vi "Autonomous Independent.vi"() -> ()   [LabVIEW 2019]
doc: "This VI is called when autonomous begins, and will automatically be terminated when autonomous ends. You can carry out timed or sensor driven robot movement independently without needing to return to the caller."
uses:
  <vilib>/Rock Robotics/WPI/Utilities/WPI_GetSetVariantRefNum.vi
  <vilib>/Rock Robotics/Network Tables/NT Read String.vi
  <vilib>/Rock Robotics/Network Tables/NT Write Numeric Array.vi
  <vilib>/Rock Robotics/Network Tables/NT Write Number.vi
  <vilib>/Rock Robotics/Network Tables/NT Write Boolean.vi
  <vilib>/Rock Robotics/WPI/RobotDrive/WPI_RobotDriveArcadeDrive_Standard(NoSaturation).vi
panel:
  out "Current Movement, for debugging":T1 {"Y Joystick Value" scale=1.0..-1.0; "X Joystick Value" scale=-1.0..1.0}
  in  "Array of robot movements":T2(array[cluster])=[{"X Joystick Value"=0.39393939393939403, "Y Joystick Value"=0.0, "Delay (sec)"=1.0, "Movement Name"="turn"}, {"X Joystick Value"=-0.3737373737373737, "Y Joystick Value"=0.0, "Delay (sec)"=1.0, "Movement Name"="turn back"}] {"Y Joystick Value" scale=1.0..-1.0; "X Joystick Value" scale=-1.0..1.0}
  # "Be sure to right-click and choose Data Operations>>Make Current Value default if you want to save the array values with the VI"
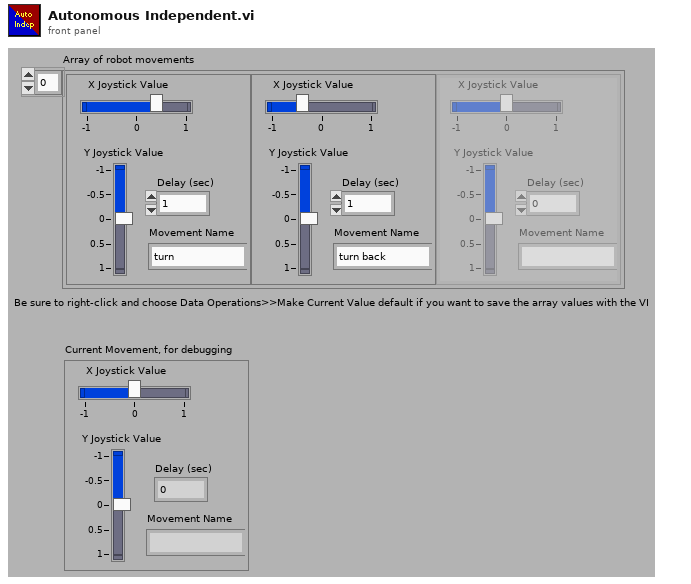
[diagram p1: front panel]
types:
  T1 = cluster{"X Joystick Value":dbl, "Y Joystick Value":dbl, "Delay (sec)":dbl, "Movement Name":string}
  T2 = cluster{"X Joystick Value":dbl, "Y Joystick Value":dbl, "Delay (sec)":dbl, "Movement Name":string}[]
  T3 = typedef "WPI_JoystickDevRef.ctl" = cluster{"Device":T4}
  T4 = typedef "WPI_JoystickDeviceEnum.ctl" = enum16{"USB 0", "USB 1", "USB 2", "USB 3", "USB 4", "USB 5"}
  T5 = typedef "WPI_ServoDeviceRef.ctl" = cluster{"DeviceStatus":errorcluster, "PWM Channel":T6, "DeadBand":T7}
  T6 = typedef "FPGA_DIOPWMChannel.ctl" = enum8{"PWM 0", "PWM 1", "PWM 2", "PWM 3", "PWM 4", "PWM 5", "PWM 6", "PWM 7", "PWM 8", "PWM 9", "PWM MXP 0", "PWM MXP 1", "PWM MXP 2", "PWM MXP 3", "PWM MXP 4", "PWM MXP 5", "PWM MXP 6", "PWM MXP 7", "PWM MXP 8", "PWM MXP 9", "Invalid"}
  T7 = typedef "WPI_PWMDeadband.ctl" = cluster{"Name":string, "maxPositivePwm":i32, "minPositivePwm":i32, "centerPwm":i32, "maxNegativePwm":i32, "minNegativePwm":i32, "angularRange":u16}
  T8 = typedef "WPI_MotorControlDeviceRef.ctl" = cluster{"DeviceStatus":errorcluster, "Type":T9, "PWM":cluster{"PWM Channel":T6, "DeadBand":T7}, "CAN":cluster{"Device Number":u8, "SetOutput VI Ref":variant, "GetOutput VI Ref":variant, "Enable VI Ref":variant, "Disable VI Ref":variant, "Data":variant}, "Invert":bool, "DIO PWM":cluster{"PWM \"Enable\" Channel":T6, "DIOChannel":T10, "PWM Rate":dbl}}
  T9 = typedef "WPI_MotorControlType.ctl" = enum16{"PWM", "CAN", "DIO PWM"}
  T10 = typedef "FPGA_DIOChannel.ctl" = enum8{"DIO 0", "DIO 1", "DIO 2", "DIO 3", "DIO 4", "DIO 5", "DIO 6", "DIO 7", "DIO 8", "DIO 9", "DIO MXP 0", "DIO MXP 1", "DIO MXP 2", "DIO MXP 3", "DIO MXP 4", "DIO MXP 5", "DIO MXP 6", "DIO MXP 7", "DIO MXP 8", "DIO MXP 9", "DIO MXP 10", "DIO MXP 11", "DIO MXP 12", "DIO MXP 13", "DIO MXP 14", "DIO MXP 15", "SPI Port CS1", "SPI Port CS2", "SPI Port CS3", "SPI Port MISO", "SPI Port MOSI", "Invalid"}
  T11 = typedef "WPI_RobotDriveDevRef.ctl" = cluster{"DevStatus":errorcluster, "Motors[]":T8[], "Square Inputs":bool, "Max Output":dbl}
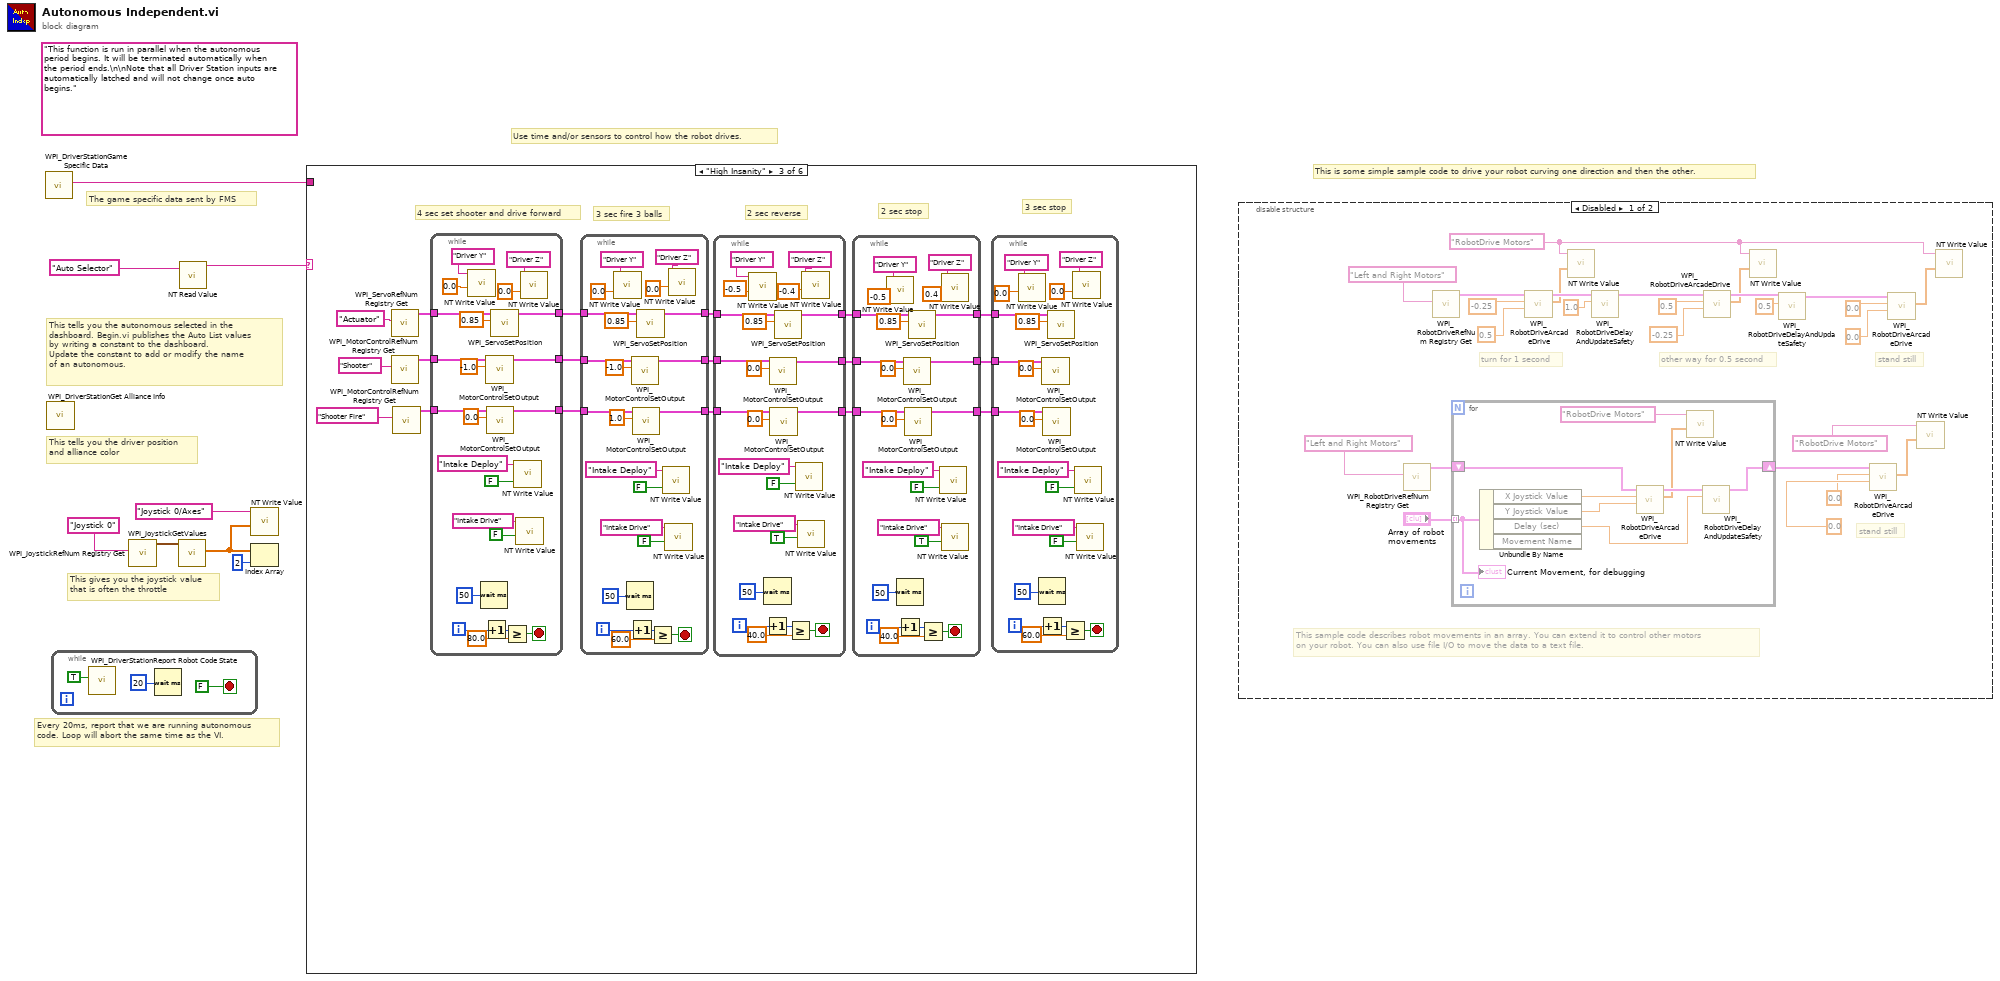
[diagram p0: block diagram]
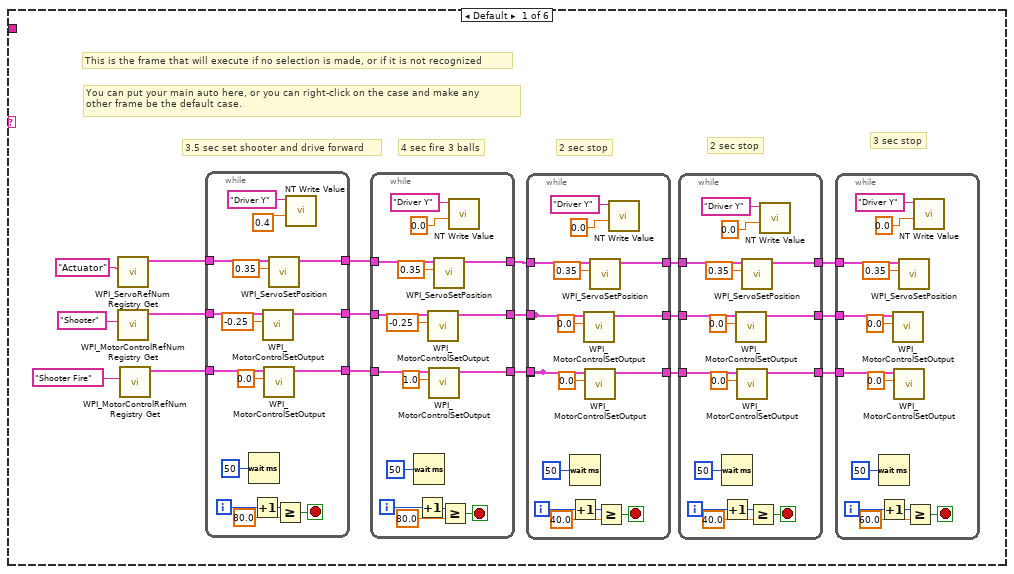
[diagram p3: hidden frame]
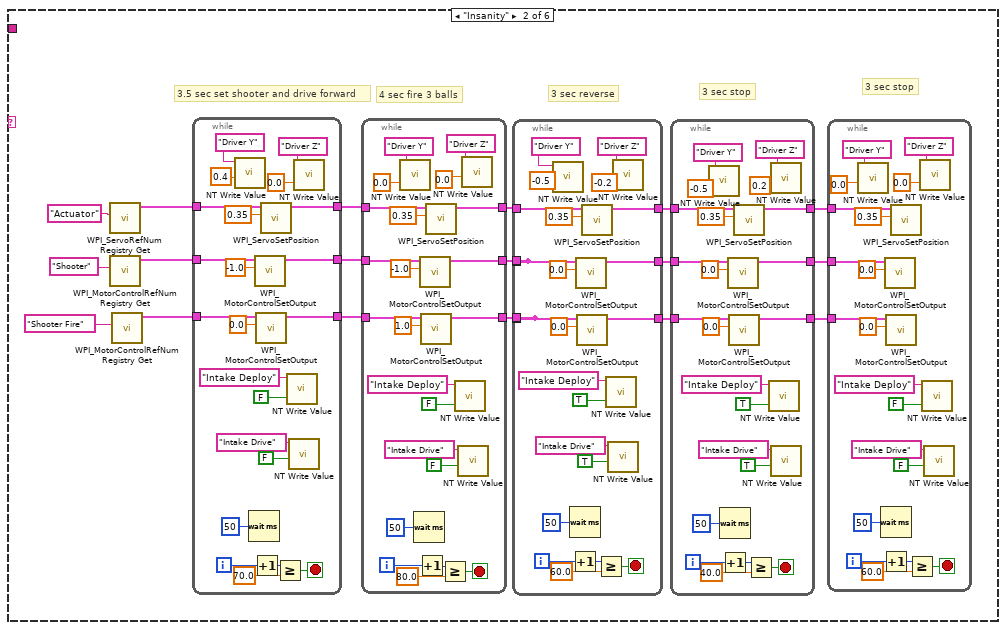
[diagram p4: hidden frame]
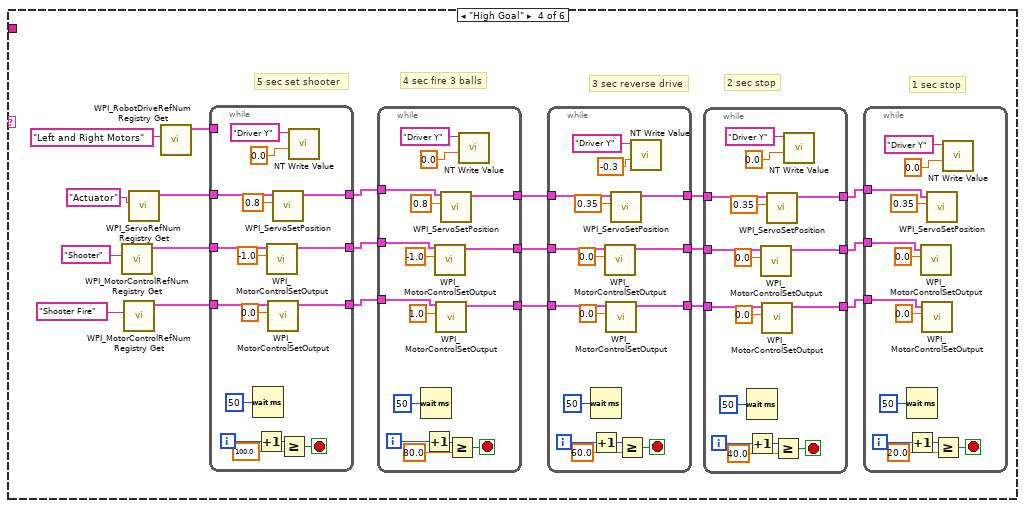
[diagram p5: hidden frame]
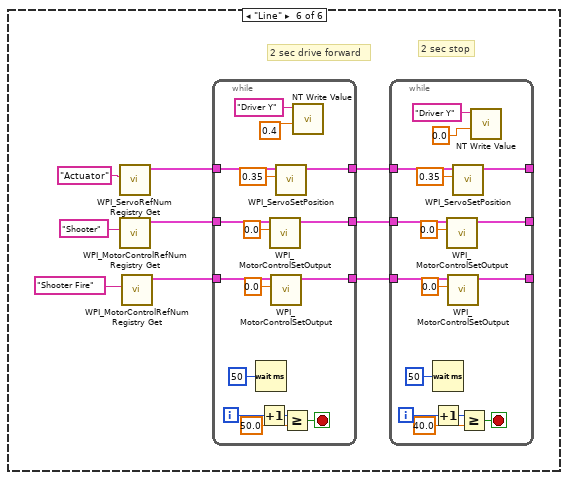
[diagram p7: hidden frame]
diagram:
  (unwired) "This function is run in parallel when the autonomous period begins. It will be terminated automatically when the period ends.\n\nNote that all Driver Station inputs are automatically latched and will not change once auto begins."
  # "This is some simple sample code to drive your robot curving one direction and then the other."
  # "The game specific data sent by FMS"
  # "This tells you the autonomous selected in the \ndashboard. Begin.vi publishes the Auto List values\nby writing a constant to the dashboard.\nUpdate the constant to add or modify the name\nof an autonomous."
  # "Every 20ms, report that we are running autonomous\ncode. Loop will abort the same time as the VI."
  # "This gives you the joystick value\nthat is often the throttle"
  # "Use time and/or sensors to control how the robot drives."
  # "This tells you the driver position\nand alliance color"
  n1 = call <vilib>:"WPI_DriverStationGame Specific Data.vi"() -> ("Game Specific Data"=w1:string)  [unwired: 11 in]
  n2 = call <vilib>:"WPI_DriverStationGet Alliance Info.vi"() -> ()  [unwired: 12 out]
  n3 = while {
    stop <- FALSE stop-if-true
    n4 = call <vilib>:"WPI_DriverStationReport Robot Code State.vi"("Autonomous"=TRUE) -> ()  [unwired: 10 in, 1 out]
    n5 = Wait (ms)(milliseconds to wait=u32 20) -> ()  [unwired: 1 out]
  }
  n6 = call <vilib>:"WPI_JoystickRefNum Registry Get.vi"("refnum name"="Joystick 0") -> ("JoystickDevRef"=w7:T3)  [unwired: 1 in, 9 out]
  n7 = call <vilib>:"WPI_JoystickGetValues.vi"("JoystickDevRef"=w7) -> ("Axes"=w3:dbl[])  [unwired: 6 in, 4 out]
  n8 = call-poly <vilib>:"NT Read Value.vi"("Name"="Auto Selector") -> ("String"=w4:string)  [unwired: 9 in, 1 out]
  n9 = call-poly <vilib>:"NT Write Value.vi"("Numeric Array"=w3, "Name"="Joystick 0/Axes") -> ()  [unwired: 9 in, 1 out]
  n10 = Index Array(array=w3, index=2) -> ()  [unwired: 1 out]
  n11 = case shown="\"High Insanity\"" w4 {
    tunnel: w1 -> [_ _ _ _ _ _]
    frame Default {
      # "2 sec stop"
      # "4 sec fire 3 balls"
      # "3 sec stop"
      # "2 sec stop"
      # "3.5 sec set shooter and drive forward"
      # "You can put your main auto here, or you can right-click on the case and make any\nother frame be the default case."
      # "This is the frame that will execute if no selection is made, or if it is not recognized"
      n12 = call <vilib>:"WPI_ServoRefNum Registry Get.vi"("refnum name"="Actuator") -> ("ServoDeviceRef"=w26:T5)  [unwired: 9 in, 1 out]
      n13 = call <vilib>:"WPI_MotorControlRefNum Registry Get.vi"("refnum name"="Shooter") -> ("MotorControlDevRef"=w25:T8)  [unwired: 9 in, 1 out]
      n14 = call <vilib>:"WPI_MotorControlRefNum Registry Get.vi"("refnum name"="Shooter Fire") -> ("MotorControlDevRef"=w24:T8)  [unwired: 9 in, 1 out]
      n15 = while {
        tunnel: w25 -> [w101]
        tunnel: w24 -> [w100]
        tunnel: w26 -> [w99]
        tunnel: [w95] -> w23
        tunnel: [w94] -> w22
        tunnel: [w93] -> w21
        i -> [w103]
        stop <- w104 stop-if-true
        n16 = Wait (ms)(milliseconds to wait=u32 50) -> ()  [unwired: 1 out]
        n17 = Increment(x=w103) -> (x+1=w102:i32)
        n18 = call <vilib>:"WPI_MotorControlSetOutput.vi"("Output"=-0.25, "MotorControlDevRef"=w101) -> ("MotorControlDevRef"=w94:T8)  [unwired: 7 in, 2 out]
        n19 = call <vilib>:"WPI_MotorControlSetOutput.vi"("Output"=0.0, "MotorControlDevRef"=w100) -> ("MotorControlDevRef"=w93:T8)  [unwired: 7 in, 2 out]
        n20 = call <vilib>:"WPI_ServoSetPosition.vi"("Position"=0.35, "ServoDeviceRef"=w99) -> ("ServoDeviceRef"=w95:T5)  [unwired: 8 in, 1 out]
        n21 = Greater Or Equal?(x=w102, y=80.0) -> (x >= y?=w104:bool)
        n22 = call-poly <vilib>:"NT Write Value.vi"("Numeric"=0.4, "Name"="Driver Y") -> ()  [unwired: 9 in, 1 out]
      }
      n23 = while {
        tunnel: w22 -> [w85]
        tunnel: w21 -> [w84]
        tunnel: w23 -> [w83]
        tunnel: [w79] -> w20
        tunnel: [w78] -> w19
        tunnel: [w77] -> w18
        i -> [w87]
        stop <- w88 stop-if-true
        n24 = Wait (ms)(milliseconds to wait=u32 50) -> ()  [unwired: 1 out]
        n25 = Increment(x=w87) -> (x+1=w86:i32)
        n26 = call <vilib>:"WPI_MotorControlSetOutput.vi"("Output"=-0.25, "MotorControlDevRef"=w85) -> ("MotorControlDevRef"=w78:T8)  [unwired: 7 in, 2 out]
        n27 = call <vilib>:"WPI_MotorControlSetOutput.vi"("Output"=1.0, "MotorControlDevRef"=w84) -> ("MotorControlDevRef"=w77:T8)  [unwired: 7 in, 2 out]
        n28 = call <vilib>:"WPI_ServoSetPosition.vi"("Position"=0.35, "ServoDeviceRef"=w83) -> ("ServoDeviceRef"=w79:T5)  [unwired: 8 in, 1 out]
        n29 = Greater Or Equal?(x=w86, y=80.0) -> (x >= y?=w88:bool)
        n30 = call-poly <vilib>:"NT Write Value.vi"("Numeric"=0.0, "Name"="Driver Y") -> ()  [unwired: 9 in, 1 out]
      }
      n31 = while {
        tunnel: [w60] -> _
        tunnel: [w59] -> _
        tunnel: w20 -> [w69]
        tunnel: [w65] -> w15
        tunnel: [w64] -> w16
        tunnel: [w63] -> w17
        tunnel: w19 -> [w60]
        tunnel: w18 -> [w59]
        i -> [w71]
        stop <- w72 stop-if-true
        n32 = Wait (ms)(milliseconds to wait=u32 50) -> ()  [unwired: 1 out]
        n33 = Increment(x=w71) -> (x+1=w70:i32)
        n34 = call <vilib>:"WPI_MotorControlSetOutput.vi"("Output"=0.0, "MotorControlDevRef"=w60) -> ("MotorControlDevRef"=w64:T8)  [unwired: 7 in, 2 out]
        n35 = call <vilib>:"WPI_MotorControlSetOutput.vi"("Output"=0.0, "MotorControlDevRef"=w59) -> ("MotorControlDevRef"=w63:T8)  [unwired: 7 in, 2 out]
        n36 = call <vilib>:"WPI_ServoSetPosition.vi"("Position"=0.35, "ServoDeviceRef"=w69) -> ("ServoDeviceRef"=w65:T5)  [unwired: 8 in, 1 out]
        n37 = Greater Or Equal?(x=w70, y=40.0) -> (x >= y?=w72:bool)
        n38 = call-poly <vilib>:"NT Write Value.vi"("Numeric"=0.0, "Name"="Driver Y") -> ()  [unwired: 9 in, 1 out]
      }
      n39 = while {
        tunnel: w16 -> [w53]
        tunnel: w17 -> [w52]
        tunnel: w15 -> [w51]
        tunnel: [w47] -> w14
        tunnel: [w46] -> w13
        tunnel: [w45] -> w12
        i -> [w55]
        stop <- w56 stop-if-true
        n40 = Wait (ms)(milliseconds to wait=u32 50) -> ()  [unwired: 1 out]
        n41 = Increment(x=w55) -> (x+1=w54:i32)
        n42 = call <vilib>:"WPI_MotorControlSetOutput.vi"("Output"=0.0, "MotorControlDevRef"=w53) -> ("MotorControlDevRef"=w46:T8)  [unwired: 7 in, 2 out]
        n43 = call <vilib>:"WPI_MotorControlSetOutput.vi"("Output"=0.0, "MotorControlDevRef"=w52) -> ("MotorControlDevRef"=w45:T8)  [unwired: 7 in, 2 out]
        n44 = call <vilib>:"WPI_ServoSetPosition.vi"("Position"=0.35, "ServoDeviceRef"=w51) -> ("ServoDeviceRef"=w47:T5)  [unwired: 8 in, 1 out]
        n45 = Greater Or Equal?(x=w54, y=40.0) -> (x >= y?=w56:bool)
        n46 = call-poly <vilib>:"NT Write Value.vi"("Numeric"=0.0, "Name"="Driver Y") -> ()  [unwired: 9 in, 1 out]
      }
      n47 = while {
        tunnel: w13 -> [w37]
        tunnel: w12 -> [w36]
        tunnel: w14 -> [w35]
        i -> [w39]
        stop <- w40 stop-if-true
        n48 = Wait (ms)(milliseconds to wait=u32 50) -> ()  [unwired: 1 out]
        n49 = Increment(x=w39) -> (x+1=w38:i32)
        n50 = call <vilib>:"WPI_MotorControlSetOutput.vi"("Output"=0.0, "MotorControlDevRef"=w37) -> ()  [unwired: 7 in, 3 out]
        n51 = call <vilib>:"WPI_MotorControlSetOutput.vi"("Output"=0.0, "MotorControlDevRef"=w36) -> ()  [unwired: 7 in, 3 out]
        n52 = call <vilib>:"WPI_ServoSetPosition.vi"("Position"=0.35, "ServoDeviceRef"=w35) -> ()  [unwired: 8 in, 2 out]
        n53 = Greater Or Equal?(x=w38, y=60.0) -> (x >= y?=w40:bool)
        n54 = call-poly <vilib>:"NT Write Value.vi"("Numeric"=0.0, "Name"="Driver Y") -> ()  [unwired: 9 in, 1 out]
      }
    }
    frame "Insanity" {
      # "3 sec reverse"
      # "4 sec fire 3 balls"
      # "3 sec stop"
      # "3 sec stop"
      # "3.5 sec set shooter and drive forward"
      n55 = call <vilib>:"WPI_ServoRefNum Registry Get.vi"("refnum name"="Actuator") -> ("ServoDeviceRef"=w121:T5)  [unwired: 9 in, 1 out]
      n56 = call <vilib>:"WPI_MotorControlRefNum Registry Get.vi"("refnum name"="Shooter") -> ("MotorControlDevRef"=w120:T8)  [unwired: 9 in, 1 out]
      n57 = call <vilib>:"WPI_MotorControlRefNum Registry Get.vi"("refnum name"="Shooter Fire") -> ("MotorControlDevRef"=w119:T8)  [unwired: 9 in, 1 out]
      n58 = while {
        tunnel: w120 -> [w226]
        tunnel: w119 -> [w225]
        tunnel: w121 -> [w224]
        tunnel: [w220] -> w118
        tunnel: [w219] -> w117
        tunnel: [w218] -> w116
        i -> [w228]
        stop <- w229 stop-if-true
        n59 = call-poly <vilib>:"NT Write Value.vi"("Numeric"=0.4, "Name"="Driver Y") -> ()  [unwired: 9 in, 1 out]
        n60 = Wait (ms)(milliseconds to wait=u32 50) -> ()  [unwired: 1 out]
        n61 = Increment(x=w228) -> (x+1=w227:i32)
        n62 = call <vilib>:"WPI_MotorControlSetOutput.vi"("Output"=-1.0, "MotorControlDevRef"=w226) -> ("MotorControlDevRef"=w219:T8)  [unwired: 7 in, 2 out]
        n63 = call <vilib>:"WPI_MotorControlSetOutput.vi"("Output"=0.0, "MotorControlDevRef"=w225) -> ("MotorControlDevRef"=w218:T8)  [unwired: 7 in, 2 out]
        n64 = call <vilib>:"WPI_ServoSetPosition.vi"("Position"=0.35, "ServoDeviceRef"=w224) -> ("ServoDeviceRef"=w220:T5)  [unwired: 8 in, 1 out]
        n65 = Greater Or Equal?(x=w227, y=70.0) -> (x >= y?=w229:bool)
        n66 = call-poly <vilib>:"NT Write Value.vi"("Boolean"=FALSE, "Name"="Intake Deploy") -> ()  [unwired: 9 in, 1 out]
        n67 = call-poly <vilib>:"NT Write Value.vi"("Boolean"=FALSE, "Name"="Intake Drive") -> ()  [unwired: 9 in, 1 out]
        n68 = call-poly <vilib>:"NT Write Value.vi"("Numeric"=0.0, "Name"="Driver Z") -> ()  [unwired: 9 in, 1 out]
      }
      n69 = while {
        tunnel: w117 -> [w204]
        tunnel: w116 -> [w203]
        tunnel: w118 -> [w202]
        tunnel: [w198] -> w115
        tunnel: [w197] -> w114
        tunnel: [w196] -> w113
        i -> [w206]
        stop <- w207 stop-if-true
        n70 = call-poly <vilib>:"NT Write Value.vi"("Numeric"=0.0, "Name"="Driver Y") -> ()  [unwired: 9 in, 1 out]
        n71 = Wait (ms)(milliseconds to wait=u32 50) -> ()  [unwired: 1 out]
        n72 = Increment(x=w206) -> (x+1=w205:i32)
        n73 = call <vilib>:"WPI_MotorControlSetOutput.vi"("Output"=-1.0, "MotorControlDevRef"=w204) -> ("MotorControlDevRef"=w197:T8)  [unwired: 7 in, 2 out]
        n74 = call <vilib>:"WPI_MotorControlSetOutput.vi"("Output"=1.0, "MotorControlDevRef"=w203) -> ("MotorControlDevRef"=w196:T8)  [unwired: 7 in, 2 out]
        n75 = call <vilib>:"WPI_ServoSetPosition.vi"("Position"=0.35, "ServoDeviceRef"=w202) -> ("ServoDeviceRef"=w198:T5)  [unwired: 8 in, 1 out]
        n76 = Greater Or Equal?(x=w205, y=80.0) -> (x >= y?=w207:bool)
        n77 = call-poly <vilib>:"NT Write Value.vi"("Boolean"=FALSE, "Name"="Intake Deploy") -> ()  [unwired: 9 in, 1 out]
        n78 = call-poly <vilib>:"NT Write Value.vi"("Boolean"=FALSE, "Name"="Intake Drive") -> ()  [unwired: 9 in, 1 out]
        n79 = call-poly <vilib>:"NT Write Value.vi"("Numeric"=0.0, "Name"="Driver Z") -> ()  [unwired: 9 in, 1 out]
      }
      n80 = while {
        tunnel: [w173] -> _
        tunnel: [w172] -> _
        tunnel: w115 -> [w182]
        tunnel: [w178] -> w110
        tunnel: [w177] -> w111
        tunnel: [w176] -> w112
        tunnel: w114 -> [w173]
        tunnel: w113 -> [w172]
        i -> [w184]
        stop <- w185 stop-if-true
        n81 = call-poly <vilib>:"NT Write Value.vi"("Numeric"=-0.5, "Name"="Driver Y") -> ()  [unwired: 9 in, 1 out]
        n82 = Wait (ms)(milliseconds to wait=u32 50) -> ()  [unwired: 1 out]
        n83 = Increment(x=w184) -> (x+1=w183:i32)
        n84 = call <vilib>:"WPI_MotorControlSetOutput.vi"("Output"=0.0, "MotorControlDevRef"=w173) -> ("MotorControlDevRef"=w177:T8)  [unwired: 7 in, 2 out]
        n85 = call <vilib>:"WPI_MotorControlSetOutput.vi"("Output"=0.0, "MotorControlDevRef"=w172) -> ("MotorControlDevRef"=w176:T8)  [unwired: 7 in, 2 out]
        n86 = call <vilib>:"WPI_ServoSetPosition.vi"("Position"=0.35, "ServoDeviceRef"=w182) -> ("ServoDeviceRef"=w178:T5)  [unwired: 8 in, 1 out]
        n87 = Greater Or Equal?(x=w183, y=60.0) -> (x >= y?=w185:bool)
        n88 = call-poly <vilib>:"NT Write Value.vi"("Boolean"=TRUE, "Name"="Intake Deploy") -> ()  [unwired: 9 in, 1 out]
        n89 = call-poly <vilib>:"NT Write Value.vi"("Boolean"=TRUE, "Name"="Intake Drive") -> ()  [unwired: 9 in, 1 out]
        n90 = call-poly <vilib>:"NT Write Value.vi"("Numeric"=-0.2, "Name"="Driver Z") -> ()  [unwired: 9 in, 1 out]
      }
      n91 = while {
        tunnel: w111 -> [w160]
        tunnel: w112 -> [w159]
        tunnel: w110 -> [w158]
        tunnel: [w154] -> w109
        tunnel: [w153] -> w108
        tunnel: [w152] -> w107
        i -> [w162]
        stop <- w163 stop-if-true
        n92 = call-poly <vilib>:"NT Write Value.vi"("Numeric"=-0.5, "Name"="Driver Y") -> ()  [unwired: 9 in, 1 out]
        n93 = Wait (ms)(milliseconds to wait=u32 50) -> ()  [unwired: 1 out]
        n94 = Increment(x=w162) -> (x+1=w161:i32)
        n95 = call <vilib>:"WPI_MotorControlSetOutput.vi"("Output"=0.0, "MotorControlDevRef"=w160) -> ("MotorControlDevRef"=w153:T8)  [unwired: 7 in, 2 out]
        n96 = call <vilib>:"WPI_MotorControlSetOutput.vi"("Output"=0.0, "MotorControlDevRef"=w159) -> ("MotorControlDevRef"=w152:T8)  [unwired: 7 in, 2 out]
        n97 = call <vilib>:"WPI_ServoSetPosition.vi"("Position"=0.35, "ServoDeviceRef"=w158) -> ("ServoDeviceRef"=w154:T5)  [unwired: 8 in, 1 out]
        n98 = Greater Or Equal?(x=w161, y=40.0) -> (x >= y?=w163:bool)
        n99 = call-poly <vilib>:"NT Write Value.vi"("Boolean"=TRUE, "Name"="Intake Deploy") -> ()  [unwired: 9 in, 1 out]
        n100 = call-poly <vilib>:"NT Write Value.vi"("Numeric"=0.2, "Name"="Driver Z") -> ()  [unwired: 9 in, 1 out]
        n101 = call-poly <vilib>:"NT Write Value.vi"("Boolean"=TRUE, "Name"="Intake Drive") -> ()  [unwired: 9 in, 1 out]
      }
      n102 = while {
        tunnel: w108 -> [w138]
        tunnel: w107 -> [w137]
        tunnel: w109 -> [w136]
        i -> [w140]
        stop <- w141 stop-if-true
        n103 = call-poly <vilib>:"NT Write Value.vi"("Numeric"=0.0, "Name"="Driver Y") -> ()  [unwired: 9 in, 1 out]
        n104 = Wait (ms)(milliseconds to wait=u32 50) -> ()  [unwired: 1 out]
        n105 = Increment(x=w140) -> (x+1=w139:i32)
        n106 = call <vilib>:"WPI_MotorControlSetOutput.vi"("Output"=0.0, "MotorControlDevRef"=w138) -> ()  [unwired: 7 in, 3 out]
        n107 = call <vilib>:"WPI_MotorControlSetOutput.vi"("Output"=0.0, "MotorControlDevRef"=w137) -> ()  [unwired: 7 in, 3 out]
        n108 = call <vilib>:"WPI_ServoSetPosition.vi"("Position"=0.35, "ServoDeviceRef"=w136) -> ()  [unwired: 8 in, 2 out]
        n109 = Greater Or Equal?(x=w139, y=60.0) -> (x >= y?=w141:bool)
        n110 = call-poly <vilib>:"NT Write Value.vi"("Numeric"=0.0, "Name"="Driver Z") -> ()  [unwired: 9 in, 1 out]
        n111 = call-poly <vilib>:"NT Write Value.vi"("Boolean"=FALSE, "Name"="Intake Deploy") -> ()  [unwired: 9 in, 1 out]
        n112 = call-poly <vilib>:"NT Write Value.vi"("Boolean"=FALSE, "Name"="Intake Drive") -> ()  [unwired: 9 in, 1 out]
      }
    }
    frame "High Insanity" {
      # "2 sec reverse"
      # "3 sec fire 3 balls"
      # "3 sec stop"
      # "2 sec stop"
      # "4 sec set shooter and drive forward"
      n113 = call <vilib>:"WPI_ServoRefNum Registry Get.vi"("refnum name"="Actuator") -> ("ServoDeviceRef"=w246:T5)  [unwired: 9 in, 1 out]
      n114 = call <vilib>:"WPI_MotorControlRefNum Registry Get.vi"("refnum name"="Shooter") -> ("MotorControlDevRef"=w245:T8)  [unwired: 9 in, 1 out]
      n115 = call <vilib>:"WPI_MotorControlRefNum Registry Get.vi"("refnum name"="Shooter Fire") -> ("MotorControlDevRef"=w244:T8)  [unwired: 9 in, 1 out]
      n116 = while {
        tunnel: w245 -> [w351]
        tunnel: w244 -> [w350]
        tunnel: w246 -> [w349]
        tunnel: [w345] -> w243
        tunnel: [w344] -> w242
        tunnel: [w343] -> w241
        i -> [w353]
        stop <- w354 stop-if-true
        n117 = call-poly <vilib>:"NT Write Value.vi"("Numeric"=0.0, "Name"="Driver Y") -> ()  [unwired: 9 in, 1 out]
        n118 = Wait (ms)(milliseconds to wait=u32 50) -> ()  [unwired: 1 out]
        n119 = Increment(x=w353) -> (x+1=w352:i32)
        n120 = call <vilib>:"WPI_MotorControlSetOutput.vi"("Output"=-1.0, "MotorControlDevRef"=w351) -> ("MotorControlDevRef"=w344:T8)  [unwired: 7 in, 2 out]
        n121 = call <vilib>:"WPI_MotorControlSetOutput.vi"("Output"=0.0, "MotorControlDevRef"=w350) -> ("MotorControlDevRef"=w343:T8)  [unwired: 7 in, 2 out]
        n122 = call <vilib>:"WPI_ServoSetPosition.vi"("Position"=0.85, "ServoDeviceRef"=w349) -> ("ServoDeviceRef"=w345:T5)  [unwired: 8 in, 1 out]
        n123 = Greater Or Equal?(x=w352, y=80.0) -> (x >= y?=w354:bool)
        n124 = call-poly <vilib>:"NT Write Value.vi"("Boolean"=FALSE, "Name"="Intake Deploy") -> ()  [unwired: 9 in, 1 out]
        n125 = call-poly <vilib>:"NT Write Value.vi"("Boolean"=FALSE, "Name"="Intake Drive") -> ()  [unwired: 9 in, 1 out]
        n126 = call-poly <vilib>:"NT Write Value.vi"("Numeric"=0.0, "Name"="Driver Z") -> ()  [unwired: 9 in, 1 out]
      }
      n127 = while {
        tunnel: w242 -> [w329]
        tunnel: w241 -> [w328]
        tunnel: w243 -> [w327]
        tunnel: [w323] -> w240
        tunnel: [w322] -> w239
        tunnel: [w321] -> w238
        i -> [w331]
        stop <- w332 stop-if-true
        n128 = call-poly <vilib>:"NT Write Value.vi"("Numeric"=0.0, "Name"="Driver Y") -> ()  [unwired: 9 in, 1 out]
        n129 = Wait (ms)(milliseconds to wait=u32 50) -> ()  [unwired: 1 out]
        n130 = Increment(x=w331) -> (x+1=w330:i32)
        n131 = call <vilib>:"WPI_MotorControlSetOutput.vi"("Output"=-1.0, "MotorControlDevRef"=w329) -> ("MotorControlDevRef"=w322:T8)  [unwired: 7 in, 2 out]
        n132 = call <vilib>:"WPI_MotorControlSetOutput.vi"("Output"=1.0, "MotorControlDevRef"=w328) -> ("MotorControlDevRef"=w321:T8)  [unwired: 7 in, 2 out]
        n133 = call <vilib>:"WPI_ServoSetPosition.vi"("Position"=0.85, "ServoDeviceRef"=w327) -> ("ServoDeviceRef"=w323:T5)  [unwired: 8 in, 1 out]
        n134 = Greater Or Equal?(x=w330, y=60.0) -> (x >= y?=w332:bool)
        n135 = call-poly <vilib>:"NT Write Value.vi"("Boolean"=FALSE, "Name"="Intake Deploy") -> ()  [unwired: 9 in, 1 out]
        n136 = call-poly <vilib>:"NT Write Value.vi"("Boolean"=FALSE, "Name"="Intake Drive") -> ()  [unwired: 9 in, 1 out]
        n137 = call-poly <vilib>:"NT Write Value.vi"("Numeric"=0.0, "Name"="Driver Z") -> ()  [unwired: 9 in, 1 out]
      }
      n138 = while {
        tunnel: w240 -> [w307]
        tunnel: [w303] -> w235
        tunnel: [w302] -> w236
        tunnel: [w301] -> w237
        tunnel: w239 -> [w291]
        tunnel: w238 -> [w292]
        i -> [w309]
        stop <- w310 stop-if-true
        n139 = call-poly <vilib>:"NT Write Value.vi"("Numeric"=-0.5, "Name"="Driver Y") -> ()  [unwired: 9 in, 1 out]
        n140 = Wait (ms)(milliseconds to wait=u32 50) -> ()  [unwired: 1 out]
        n141 = Increment(x=w309) -> (x+1=w308:i32)
        n142 = call <vilib>:"WPI_MotorControlSetOutput.vi"("Output"=0.0, "MotorControlDevRef"=w291) -> ("MotorControlDevRef"=w302:T8)  [unwired: 7 in, 2 out]
        n143 = call <vilib>:"WPI_MotorControlSetOutput.vi"("Output"=0.0, "MotorControlDevRef"=w292) -> ("MotorControlDevRef"=w301:T8)  [unwired: 7 in, 2 out]
        n144 = call <vilib>:"WPI_ServoSetPosition.vi"("Position"=0.85, "ServoDeviceRef"=w307) -> ("ServoDeviceRef"=w303:T5)  [unwired: 8 in, 1 out]
        n145 = Greater Or Equal?(x=w308, y=40.0) -> (x >= y?=w310:bool)
        n146 = call-poly <vilib>:"NT Write Value.vi"("Boolean"=FALSE, "Name"="Intake Deploy") -> ()  [unwired: 9 in, 1 out]
        n147 = call-poly <vilib>:"NT Write Value.vi"("Boolean"=TRUE, "Name"="Intake Drive") -> ()  [unwired: 9 in, 1 out]
        n148 = call-poly <vilib>:"NT Write Value.vi"("Numeric"=-0.4, "Name"="Driver Z") -> ()  [unwired: 9 in, 1 out]
      }
      n149 = while {
        tunnel: w236 -> [w285]
        tunnel: w237 -> [w284]
        tunnel: w235 -> [w283]
        tunnel: [w279] -> w234
        tunnel: [w278] -> w233
        tunnel: [w277] -> w232
        i -> [w287]
        stop <- w288 stop-if-true
        n150 = call-poly <vilib>:"NT Write Value.vi"("Numeric"=-0.5, "Name"="Driver Y") -> ()  [unwired: 9 in, 1 out]
        n151 = Wait (ms)(milliseconds to wait=u32 50) -> ()  [unwired: 1 out]
        n152 = Increment(x=w287) -> (x+1=w286:i32)
        n153 = call <vilib>:"WPI_MotorControlSetOutput.vi"("Output"=0.0, "MotorControlDevRef"=w285) -> ("MotorControlDevRef"=w278:T8)  [unwired: 7 in, 2 out]
        n154 = call <vilib>:"WPI_MotorControlSetOutput.vi"("Output"=0.0, "MotorControlDevRef"=w284) -> ("MotorControlDevRef"=w277:T8)  [unwired: 7 in, 2 out]
        n155 = call <vilib>:"WPI_ServoSetPosition.vi"("Position"=0.85, "ServoDeviceRef"=w283) -> ("ServoDeviceRef"=w279:T5)  [unwired: 8 in, 1 out]
        n156 = Greater Or Equal?(x=w286, y=40.0) -> (x >= y?=w288:bool)
        n157 = call-poly <vilib>:"NT Write Value.vi"("Boolean"=FALSE, "Name"="Intake Deploy") -> ()  [unwired: 9 in, 1 out]
        n158 = call-poly <vilib>:"NT Write Value.vi"("Numeric"=0.4, "Name"="Driver Z") -> ()  [unwired: 9 in, 1 out]
        n159 = call-poly <vilib>:"NT Write Value.vi"("Boolean"=TRUE, "Name"="Intake Drive") -> ()  [unwired: 9 in, 1 out]
      }
      n160 = while {
        tunnel: w233 -> [w263]
        tunnel: w232 -> [w262]
        tunnel: w234 -> [w261]
        i -> [w265]
        stop <- w266 stop-if-true
        n161 = call-poly <vilib>:"NT Write Value.vi"("Numeric"=0.0, "Name"="Driver Y") -> ()  [unwired: 9 in, 1 out]
        n162 = Wait (ms)(milliseconds to wait=u32 50) -> ()  [unwired: 1 out]
        n163 = Increment(x=w265) -> (x+1=w264:i32)
        n164 = call <vilib>:"WPI_MotorControlSetOutput.vi"("Output"=0.0, "MotorControlDevRef"=w263) -> ()  [unwired: 7 in, 3 out]
        n165 = call <vilib>:"WPI_MotorControlSetOutput.vi"("Output"=0.0, "MotorControlDevRef"=w262) -> ()  [unwired: 7 in, 3 out]
        n166 = call <vilib>:"WPI_ServoSetPosition.vi"("Position"=0.85, "ServoDeviceRef"=w261) -> ()  [unwired: 8 in, 2 out]
        n167 = Greater Or Equal?(x=w264, y=60.0) -> (x >= y?=w266:bool)
        n168 = call-poly <vilib>:"NT Write Value.vi"("Numeric"=0.0, "Name"="Driver Z") -> ()  [unwired: 9 in, 1 out]
        n169 = call-poly <vilib>:"NT Write Value.vi"("Boolean"=FALSE, "Name"="Intake Deploy") -> ()  [unwired: 9 in, 1 out]
        n170 = call-poly <vilib>:"NT Write Value.vi"("Boolean"=FALSE, "Name"="Intake Drive") -> ()  [unwired: 9 in, 1 out]
      }
    }
    frame "High Goal" {
      # "1 sec stop"
      # "2 sec stop"
      # "4 sec fire 3 balls"
      # "3 sec reverse drive"
      # "5 sec set shooter"
      n171 = call <vilib>:"WPI_MotorControlRefNum Registry Get.vi"("refnum name"="Shooter") -> ("MotorControlDevRef"=w374:T8)  [unwired: 9 in, 1 out]
      n172 = call <vilib>:"WPI_MotorControlRefNum Registry Get.vi"("refnum name"="Shooter Fire") -> ("MotorControlDevRef"=w371:T8)  [unwired: 9 in, 1 out]
      n173 = call <vilib>:"WPI_ServoRefNum Registry Get.vi"("refnum name"="Actuator") -> ("ServoDeviceRef"=w369:T5)  [unwired: 9 in, 1 out]
      n174 = call <vilib>:"WPI_RobotDriveRefNum Registry Get.vi"("refnum name"="Left and Right Motors") -> ("RobotDriveDevRef"=w373:T11)  [unwired: 1 in, 9 out]
      n175 = while {
        tunnel: w374 -> [w448]
        tunnel: w373 -> [_]
        tunnel: w371 -> [w447]
        tunnel: w369 -> [w446]
        tunnel: [w442] -> w368
        tunnel: [w441] -> w367
        tunnel: [w440] -> w366
        i -> [w450]
        stop <- w451 stop-if-true
        n176 = Wait (ms)(milliseconds to wait=u32 50) -> ()  [unwired: 1 out]
        n177 = Increment(x=w450) -> (x+1=w449:i32)
        n178 = call <vilib>:"WPI_MotorControlSetOutput.vi"("Output"=-1.0, "MotorControlDevRef"=w448) -> ("MotorControlDevRef"=w441:T8)  [unwired: 7 in, 2 out]
        n179 = call <vilib>:"WPI_MotorControlSetOutput.vi"("Output"=0.0, "MotorControlDevRef"=w447) -> ("MotorControlDevRef"=w440:T8)  [unwired: 7 in, 2 out]
        n180 = call <vilib>:"WPI_ServoSetPosition.vi"("Position"=0.8, "ServoDeviceRef"=w446) -> ("ServoDeviceRef"=w442:T5)  [unwired: 8 in, 1 out]
        n181 = Greater Or Equal?(x=w449, y=100.0) -> (x >= y?=w451:bool)
        n182 = call-poly <vilib>:"NT Write Value.vi"("Numeric"=0.0, "Name"="Driver Y") -> ()  [unwired: 9 in, 1 out]
      }
      n183 = while {
        tunnel: [w400] -> w365
        tunnel: [w399] -> w364
        tunnel: [w398] -> w363
        tunnel: w368 -> [w397]
        tunnel: w367 -> [w396]
        tunnel: w366 -> [w395]
        i -> [w405]
        stop <- w406 stop-if-true
        n184 = Wait (ms)(milliseconds to wait=u32 50) -> ()  [unwired: 1 out]
        n185 = Increment(x=w405) -> (x+1=w404:i32)
        n186 = call <vilib>:"WPI_MotorControlSetOutput.vi"("Output"=-1.0, "MotorControlDevRef"=w396) -> ("MotorControlDevRef"=w399:T8)  [unwired: 7 in, 2 out]
        n187 = call <vilib>:"WPI_MotorControlSetOutput.vi"("Output"=1.0, "MotorControlDevRef"=w395) -> ("MotorControlDevRef"=w398:T8)  [unwired: 7 in, 2 out]
        n188 = call <vilib>:"WPI_ServoSetPosition.vi"("Position"=0.8, "ServoDeviceRef"=w397) -> ("ServoDeviceRef"=w400:T5)  [unwired: 8 in, 1 out]
        n189 = Greater Or Equal?(x=w404, y=80.0) -> (x >= y?=w406:bool)
        n190 = call-poly <vilib>:"NT Write Value.vi"("Numeric"=0.0, "Name"="Driver Y") -> ()  [unwired: 9 in, 1 out]
      }
      n191 = while {
        tunnel: w364 -> [w432]
        tunnel: w363 -> [w431]
        tunnel: w365 -> [w430]
        tunnel: [w426] -> w360
        tunnel: [w425] -> w361
        tunnel: [w424] -> w362
        i -> [w434]
        stop <- w435 stop-if-true
        n192 = Wait (ms)(milliseconds to wait=u32 50) -> ()  [unwired: 1 out]
        n193 = Increment(x=w434) -> (x+1=w433:i32)
        n194 = call <vilib>:"WPI_MotorControlSetOutput.vi"("Output"=0.0, "MotorControlDevRef"=w432) -> ("MotorControlDevRef"=w425:T8)  [unwired: 7 in, 2 out]
        n195 = call <vilib>:"WPI_MotorControlSetOutput.vi"("Output"=0.0, "MotorControlDevRef"=w431) -> ("MotorControlDevRef"=w424:T8)  [unwired: 7 in, 2 out]
        n196 = call <vilib>:"WPI_ServoSetPosition.vi"("Position"=0.35, "ServoDeviceRef"=w430) -> ("ServoDeviceRef"=w426:T5)  [unwired: 8 in, 1 out]
        n197 = Greater Or Equal?(x=w433, y=60.0) -> (x >= y?=w435:bool)
        n198 = call-poly <vilib>:"NT Write Value.vi"("Numeric"=-0.3, "Name"="Driver Y") -> ()  [unwired: 9 in, 1 out]
      }
      n199 = while {
        tunnel: w361 -> [w387]
        tunnel: w362 -> [w386]
        tunnel: w360 -> [w385]
        tunnel: [w381] -> w359
        tunnel: [w380] -> w358
        tunnel: [w379] -> w357
        i -> [w389]
        stop <- w390 stop-if-true
        n200 = Wait (ms)(milliseconds to wait=u32 50) -> ()  [unwired: 1 out]
        n201 = Increment(x=w389) -> (x+1=w388:i32)
        n202 = call <vilib>:"WPI_MotorControlSetOutput.vi"("Output"=0.0, "MotorControlDevRef"=w387) -> ("MotorControlDevRef"=w380:T8)  [unwired: 7 in, 2 out]
        n203 = call <vilib>:"WPI_MotorControlSetOutput.vi"("Output"=0.0, "MotorControlDevRef"=w386) -> ("MotorControlDevRef"=w379:T8)  [unwired: 7 in, 2 out]
        n204 = call <vilib>:"WPI_ServoSetPosition.vi"("Position"=0.35, "ServoDeviceRef"=w385) -> ("ServoDeviceRef"=w381:T5)  [unwired: 8 in, 1 out]
        n205 = Greater Or Equal?(x=w388, y=40.0) -> (x >= y?=w390:bool)
        n206 = call-poly <vilib>:"NT Write Value.vi"("Numeric"=0.0, "Name"="Driver Y") -> ()  [unwired: 9 in, 1 out]
      }
      n207 = while {
        tunnel: w359 -> [w411]
        tunnel: w358 -> [w410]
        tunnel: w357 -> [w409]
        i -> [w418]
        stop <- w419 stop-if-true
        n208 = Wait (ms)(milliseconds to wait=u32 50) -> ()  [unwired: 1 out]
        n209 = Increment(x=w418) -> (x+1=w417:i32)
        n210 = call <vilib>:"WPI_MotorControlSetOutput.vi"("Output"=0.0, "MotorControlDevRef"=w410) -> ()  [unwired: 7 in, 3 out]
        n211 = call <vilib>:"WPI_MotorControlSetOutput.vi"("Output"=0.0, "MotorControlDevRef"=w409) -> ()  [unwired: 7 in, 3 out]
        n212 = call <vilib>:"WPI_ServoSetPosition.vi"("Position"=0.35, "ServoDeviceRef"=w411) -> ()  [unwired: 8 in, 2 out]
        n213 = Greater Or Equal?(x=w417, y=20.0) -> (x >= y?=w419:bool)
        n214 = call-poly <vilib>:"NT Write Value.vi"("Numeric"=0.0, "Name"="Driver Y") -> ()  [unwired: 9 in, 1 out]
      }
    }
    frame "Nothin" {
    }
    frame "Line" {
      # "2 sec drive forward"
      # "2 sec stop"
      n215 = call <vilib>:"WPI_ServoRefNum Registry Get.vi"("refnum name"="Actuator") -> ("ServoDeviceRef"=w458:T5)  [unwired: 9 in, 1 out]
      n216 = call <vilib>:"WPI_MotorControlRefNum Registry Get.vi"("refnum name"="Shooter") -> ("MotorControlDevRef"=w459:T8)  [unwired: 9 in, 1 out]
      n217 = call <vilib>:"WPI_MotorControlRefNum Registry Get.vi"("refnum name"="Shooter Fire") -> ("MotorControlDevRef"=w457:T8)  [unwired: 9 in, 1 out]
      n218 = while {
        tunnel: w459 -> [w489]
        tunnel: w457 -> [w488]
        tunnel: w458 -> [w487]
        tunnel: [w483] -> w456
        tunnel: [w482] -> w455
        tunnel: [w481] -> w454
        i -> [w491]
        stop <- w492 stop-if-true
        n219 = Wait (ms)(milliseconds to wait=u32 50) -> ()  [unwired: 1 out]
        n220 = Increment(x=w491) -> (x+1=w490:i32)
        n221 = call <vilib>:"WPI_MotorControlSetOutput.vi"("Output"=0.0, "MotorControlDevRef"=w489) -> ("MotorControlDevRef"=w482:T8)  [unwired: 7 in, 2 out]
        n222 = call <vilib>:"WPI_MotorControlSetOutput.vi"("Output"=0.0, "MotorControlDevRef"=w488) -> ("MotorControlDevRef"=w481:T8)  [unwired: 7 in, 2 out]
        n223 = call <vilib>:"WPI_ServoSetPosition.vi"("Position"=0.35, "ServoDeviceRef"=w487) -> ("ServoDeviceRef"=w483:T5)  [unwired: 8 in, 1 out]
        n224 = Greater Or Equal?(x=w490, y=50.0) -> (x >= y?=w492:bool)
        n225 = call-poly <vilib>:"NT Write Value.vi"("Numeric"=0.4, "Name"="Driver Y") -> ()  [unwired: 9 in, 1 out]
      }
      n226 = while {
        tunnel: w455 -> [w473]
        tunnel: w454 -> [w472]
        tunnel: w456 -> [w471]
        tunnel: [w467] -> _
        tunnel: [w466] -> _
        tunnel: [w465] -> _
        i -> [w475]
        stop <- w476 stop-if-true
        n227 = Wait (ms)(milliseconds to wait=u32 50) -> ()  [unwired: 1 out]
        n228 = Increment(x=w475) -> (x+1=w474:i32)
        n229 = call <vilib>:"WPI_MotorControlSetOutput.vi"("Output"=0.0, "MotorControlDevRef"=w473) -> ("MotorControlDevRef"=w466:T8)  [unwired: 7 in, 2 out]
        n230 = call <vilib>:"WPI_MotorControlSetOutput.vi"("Output"=0.0, "MotorControlDevRef"=w472) -> ("MotorControlDevRef"=w465:T8)  [unwired: 7 in, 2 out]
        n231 = call <vilib>:"WPI_ServoSetPosition.vi"("Position"=0.35, "ServoDeviceRef"=w471) -> ("ServoDeviceRef"=w467:T5)  [unwired: 8 in, 1 out]
        n232 = Greater Or Equal?(x=w474, y=40.0) -> (x >= y?=w476:bool)
        n233 = call-poly <vilib>:"NT Write Value.vi"("Numeric"=0.0, "Name"="Driver Y") -> ()  [unwired: 9 in, 1 out]
      }
    }
  }
  n234 = disable-structure shown="Disabled" {
    frame Disabled {
      w504 = "RobotDrive Motors" ("Name")
      # "stand still"
      # "This sample code describes robot movements in an array. You can extend it to control other motors\non your robot. You can also use file I/O to move the data to a text file."
      # "stand still"
      # "other way for 0.5 second"
      # "turn for 1 second"
      n235 = call <vilib>:"WPI_RobotDriveRefNum Registry Get.vi"("refnum name"="Left and Right Motors") -> ("RobotDriveDevRef"=w499:T11)  [unwired: 1 in, 9 out]
      n236 = call <vilib>:"WPI_RobotDriveRefNum Registry Get.vi"("refnum name"="Left and Right Motors") -> ("RobotDriveDevRef"=w520:T11)  [unwired: 1 in, 9 out]
      n237 = for {
        shift-right: [w527] -> w502
        shift-left: w499 -> [w528]
        tunnel: "Array of robot movements" -> [w523] mode=indexing
        n238 = Unbundle By Name(w523) -> ("X Joystick Value"=w526:dbl, "Y Joystick Value"=w525:dbl, "Delay (sec)"=w524:dbl)  [unwired: 1 out]
        n239 = call-poly <vilib>:"WPI_RobotDriveArcadeDrive.vi"("Y axis value"=w525, "X axis value"=w526, "RobotDriveDevRef"=w528) -> ("Motor Values"=w521:dbl[], "RobotDriveDevRef"=w529:T11)  [unwired: 1 in, 6 out]
        n240 = call-poly <vilib>:"NT Write Value.vi"("Numeric Array"=w521, "Name"="RobotDrive Motors") -> ()  [unwired: 9 in, 1 out]
        n241 = call <vilib>:"WPI_RobotDriveDelayAndUpdateSafety.vi"("Delay (s)"=w524, "RobotDriveDevRef"=w529) -> ("RobotDriveDevRef 2"=w527:T11)  [unwired: 8 in, 1 out]
        "Current Movement, for debugging" <- w523
      }
      n242 = call-poly <vilib>:"WPI_RobotDriveArcadeDrive.vi"("Y axis value"=0.5 ("X axis value"), "X axis value"=-0.25, "RobotDriveDevRef"=w520) -> ("Motor Values"=w503:dbl[], "RobotDriveDevRef"=w513:T11)  [unwired: 1 in, 6 out]
      n243 = call-poly <vilib>:"NT Write Value.vi"("Numeric Array"=w503, "Name"=w504) -> ()  [unwired: 9 in, 1 out]
      n244 = call <vilib>:"WPI_RobotDriveDelayAndUpdateSafety.vi"("Delay (s)"=1.0, "RobotDriveDevRef"=w513) -> ("RobotDriveDevRef 2"=w514:T11)  [unwired: 8 in, 1 out]
      n245 = call-poly <vilib>:"WPI_RobotDriveArcadeDrive.vi"("Y axis value"=-0.25 ("X axis value"), "X axis value"=0.5, "RobotDriveDevRef"=w514) -> ("Motor Values"=w505:dbl[], "RobotDriveDevRef"=w515:T11)  [unwired: 1 in, 6 out]
      n246 = call-poly <vilib>:"NT Write Value.vi"("Numeric Array"=w505, "Name"=w504) -> ()  [unwired: 9 in, 1 out]
      n247 = call <vilib>:"WPI_RobotDriveDelayAndUpdateSafety.vi"("Delay (s)"=0.5, "RobotDriveDevRef"=w515) -> ("RobotDriveDevRef 2"=w516:T11)  [unwired: 8 in, 1 out]
      n248 = call-poly <vilib>:"WPI_RobotDriveArcadeDrive.vi"("Y axis value"=0.0 ("X axis value"), "X axis value"=0.0, "RobotDriveDevRef"=w502) -> ("Motor Values"=w501:dbl[])  [unwired: 1 in, 7 out]
      n249 = call-poly <vilib>:"WPI_RobotDriveArcadeDrive.vi"("Y axis value"=0.0 ("X axis value"), "X axis value"=0.0, "RobotDriveDevRef"=w516) -> ("Motor Values"=w506:dbl[])  [unwired: 1 in, 7 out]
      n250 = call-poly <vilib>:"NT Write Value.vi"("Numeric Array"=w501, "Name"="RobotDrive Motors") -> ()  [unwired: 9 in, 1 out]
      n251 = call-poly <vilib>:"NT Write Value.vi"("Numeric Array"=w506, "Name"=w504) -> ()  [unwired: 9 in, 1 out]
    }
    frame Enabled {
    }
  }
